vi "MB Ethernet Example Slave.vi"() -> ()   [LabVIEW 2021, in "NI_modbus_upd.lvlib"]
uses:
  NI_modbus_upd.lvlib
  Ctl/Data Reference.ctl
  MB Globals.vi
  <vilib>/Analysis/NI_AALBase.lvlib
  Counter/Counter.lvlib
panel:
  out "Data Reference":T1
  in  "Listening Port":u16=502
  in  "Stop":bool
  out "Holding Registers":u16[](array[numeric]) caption="Holding Registers (Master can write in these registers)"
  out "Coils":bool[](array[boolean]) caption="Coils (Master can write coils)"
  in  "Discrete Inputs":bool[](array[boolean])=[FALSE, FALSE, FALSE, FALSE, FALSE, FALSE] caption="Discrete Inputs (Master can only read them)"
  in  "Input Registers":u16[](array[numeric]) caption="Input Registers (Master can only read them)"
  # "MB Ethernet Example Slave.vi\n\nInstructions\n1. Run this VI first (Slave/Server)\n2. Open and run MB Ethernet Example Master.vi\n3. Modify the discrete inputs or input registers on the slave -> they're updated on the master.\n4. Modify the coils and registers on the master -> they're updated on the slave."
  # "Slave Registers"
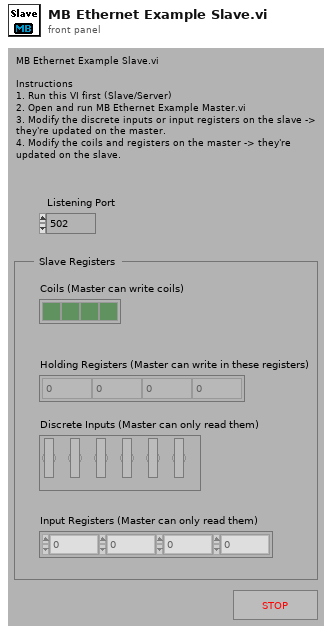
[diagram p1: front panel]
types:
  T1 = typedef "NI_modbus_upd.lvlib/Data Reference.ctl" = cluster{"DI":refnum<data-value>, "Coils":refnum<data-value>, "IR":refnum<data-value>, "HR":refnum<data-value>, "ES":refnum<data-value>, "Initialised":bool}
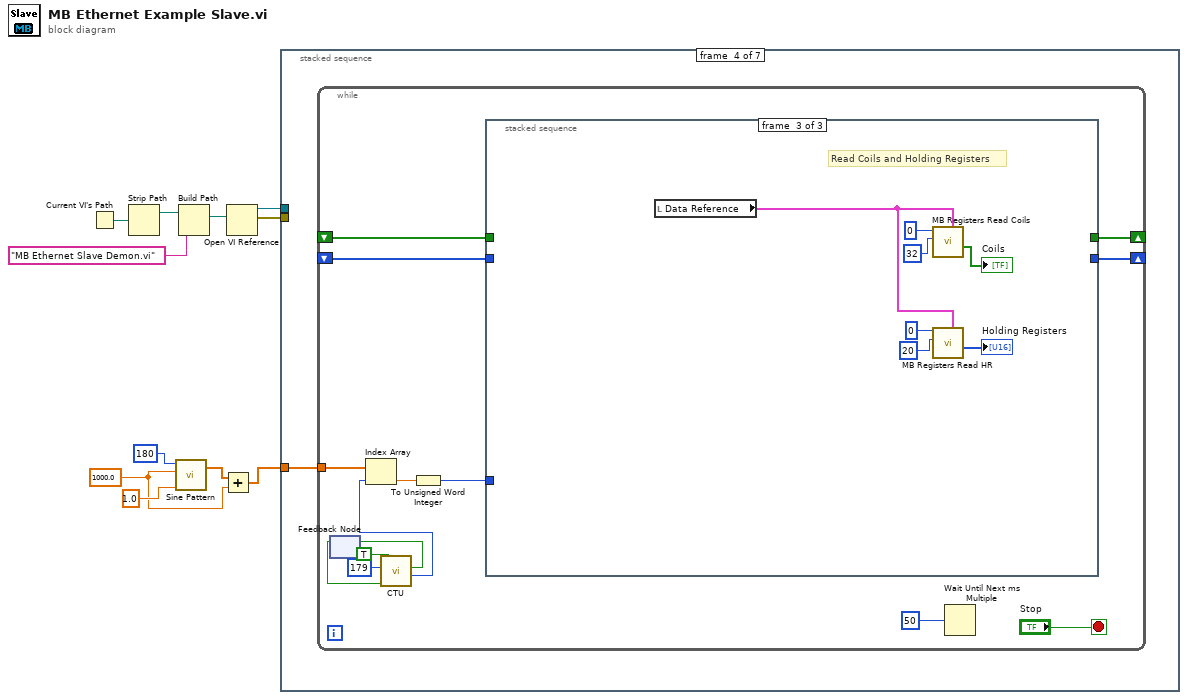
[diagram p0: block diagram]
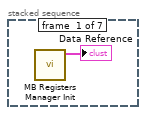
[diagram p2: hidden frame]
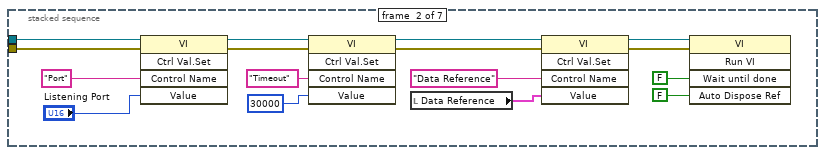
[diagram p3: hidden frame]
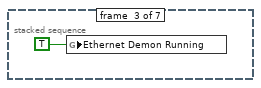
[diagram p4: hidden frame]
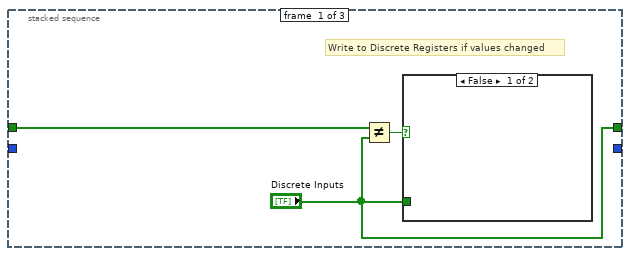
[diagram p5: hidden frame]
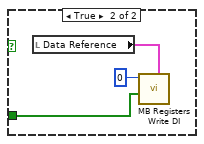
[diagram p6: hidden frame]
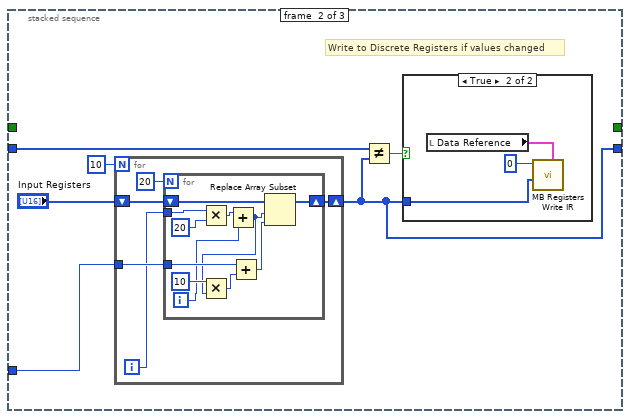
[diagram p7: hidden frame]
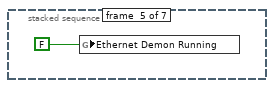
[diagram p9: hidden frame]
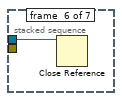
[diagram p10: hidden frame]
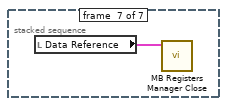
[diagram p11: hidden frame]
diagram:
  w2 = 1000.0 ("amplitude")
  n1 = Current VI's Path() -> (path=w11:path)
  n2 = Strip Path(path=w11) -> (stripped path=w10:path)  [unwired: 1 out]
  n3 = call <vilib>:"Sine Pattern.vi"("cycles"=1.0, "amplitude"=w2, "samples"=180) -> ("Sinusoidal Pattern"=w3:dbl[])  [unwired: 1 in, 1 out]
  n4 = Build Path(base path=w10, name or relative path="MB Ethernet Slave Demon.vi") -> (appended path=w8:path)
  n5 = Add(x=w3, y=w2) -> (x+y=w1:dbl[])
  n6 = Open VI Reference(vi path=w8) -> (vi reference=w7:refnum<vi>, error out=w6:errorcluster)  [unwired: 5 in]
  n7 = stacked-sequence {
    tunnel: w7 -> [_ w28 _ _ _ w84 _]
    tunnel: w6 -> [_ w27 _ _ _ _ _]
    tunnel: w1 -> [_ _ _ w30 _ _ _]
    frame #0 {
      n8 = call "MB Registers Manager Init.vi"() -> ("Data Reference"=→"Data Reference":T1)  [unwired: 10 in, 1 out]
    }
    frame #1 {
      n9 = invoke class="VI" method="Ctrl Val.Set"(reference=w28, error in=w27, "Control Name"="Port", "Value"="Listening Port") -> (reference out=w22:refnum<vi>, error out=w21:errorcluster)  [unwired: 1 in, 3 out]
      n10 = invoke class="VI" method="Ctrl Val.Set"(reference=w22, error in=w21, "Control Name"="Timeout", "Value"=u32 30000 ("Timeout")) -> (reference out=w19:refnum<vi>, error out=w18:errorcluster)  [unwired: 1 in, 3 out]
      n11 = local read "Data Reference"() -> (w17:T1)
      n12 = invoke class="VI" method="Ctrl Val.Set"(reference=w19, error in=w18, "Control Name"="Data Reference", "Value"=w17) -> (reference out=w14:refnum<vi>, error out=w13:errorcluster)  [unwired: 1 in, 3 out]
      n13 = invoke class="VI" method="Run VI"(reference=w14, error in=w13, "Wait until done"=FALSE, "Auto Dispose Ref"=FALSE) -> ()  [unwired: 1 in, 5 out]
    }
    frame #2 {
      n14 = global write "MB Globals.vi" "Ethernet Demon Running"(TRUE ("Slave Demon Running")) -> ()
    }
    frame #3 {
      n15 = while {
        shift-right: [w43] -> _
        shift-left: _ -> [w42]
        shift-right: [w40] -> _
        shift-left: _ -> [w41]
        tunnel: w30 -> [w38]
        stop <- "Stop" stop-if-true
        n16 = feedback #1() -> (w31:bool)  [unwired: 1 in]
        n17 = call "CTU.vi"("R"=w31, "DI"=u32 179, "IN"=TRUE) -> ("DO"=w34:u32, "EU"=w32:bool)  [unwired: 3 in]
        n18 = feedback-in #1(w32) -> ()
        n19 = Index Array(array=w38, index=w34) -> (element=w37:dbl)
        n20 = To Unsigned Word Integer(number=w37) -> (unsigned 16bit integer=w36:u16)
        n21 = stacked-sequence {
          tunnel: ["Discrete Inputs" _ _] -> w43
          tunnel: w42 -> [w47 _ _]
          tunnel: w41 -> [_ w55 _]
          tunnel: [_ w53 _] -> w40
          tunnel: w36 -> [_ w52 _]
          frame #0 {
            # "Write to Discrete Registers if values changed"
            n22 = Not Equal?(x=w47, y="Discrete Inputs") -> (x != y?=w45:bool)
            n23 = case shown="False" w45 {
              tunnel: "Discrete Inputs" -> [_ w49]
              frame False {
              }
              frame True {
                n24 = local read "Data Reference"() -> (w48:T1)
                n25 = call "MB Registers Write DI.vi"("Data Reference"=w48, "Bits In"=w49, "Start Address"=u16 0) -> ()  [unwired: 8 in, 1 out]
              }
            }
          }
          frame #1 {
            # "Write to Discrete Registers if values changed"
            n26 = for {
              N: 10 -> [_]
              tunnel: w52 -> [w58]
              shift-right: [w59] -> w53
              shift-left: "Input Registers" -> [w60]
              i -> [w57]
              n27 = for {
                N: 20 -> [_]
                tunnel: w58 -> [w69]
                shift-right: [w70] -> w59
                shift-left: w60 -> [w71]
                tunnel: w57 -> [w64]
                i -> [w67]
                n28 = Multiply(x=w64, y=20) -> (x*y=w65:i32)
                n29 = Add(x=w65, y=w67) -> (x+y=w62:i32)
                n30 = Multiply(x=10, y=w62) -> (x*y=w66:i32)
                n31 = Add(x=w69, y=w66) -> (x+y=w68:i32)
                n32 = Replace Array Subset(array=w71, new element=w68, index=w62) -> (w70:u16[])
              }
            }
            n33 = Not Equal?(x=w55, y=w53) -> (x != y?=w56:bool)
            n34 = case shown="True" w56 {
              tunnel: w53 -> [_ w74]
              frame False {
              }
              frame True {
                n35 = local read "Data Reference"() -> (w73:T1)
                n36 = call "MB Registers Write IR.vi"("Data Reference"=w73, "Words In"=w74, "Start Address"=u16 0) -> ()  [unwired: 8 in, 1 out]
              }
            }
          }
          frame #2 {
            # "Read Coils and Holding Registers"
            n37 = local read "Data Reference"() -> (w78:T1)
            n38 = call "MB Registers Read Coils.vi"("Data Reference"=w78, "Length"=u16 32, "Start Address"=u16 0) -> ("Bits out"=→"Coils":bool[])  [unwired: 7 in, 1 out]
            n39 = call "MB Registers Read HR.vi"("Data Reference"=w78, "Length"=u16 20, "Start Address"=u16 0) -> ("Words out"=→"Holding Registers":u16[])  [unwired: 7 in, 1 out]
          }
        }
        n40 = Wait Until Next ms Multiple(millisecond multiple=u32 50) -> ()  [unwired: 1 out]
      }
    }
    frame #4 {
      n41 = global write "MB Globals.vi" "Ethernet Demon Running"(FALSE ("Slave Demon Running")) -> ()
    }
    frame #5 {
      n42 = Close Reference(reference=w84) -> ()  [unwired: 1 in, 1 out]
    }
    frame #6 {
      n43 = local read "Data Reference"() -> (w85:T1)
      n44 = call "MB Registers Manager Close.vi"("Data Reference"=w85) -> ()  [unwired: 10 in, 1 out]
    }
  }
